vi "CRYImp wiz p4 curve select.vi"(6 "x-y settings array":T1 {"yp db ref" format="%.2f"; "ym db ref" format="%.2f"; "x db ref" format="%.2f"}, 8 "error in (no error)":errorcluster, 9 "Data in":string[][](array[string]), 10 "Main info cluster":T3, 11 "Page flags":T2) -> (0 "error out":errorcluster, 1 "Data out":string[][](array[string]), 2 "Main info cluster out":T3, 3 "Page flags out":T2, 4 "x-y settings array out":T1 {"yp db ref" format="%.2f"; "ym db ref" format="%.2f"; "x db ref" format="%.2f"}, 5 "Data array out":string[](array[string]))   [LabVIEW 2013]
uses:
  Control/CRYImp wiz page flags.ctl
  Control/CRYImp wiz main info.ctl
  Control/CRYx-y settings array.ctl
  CRYImp wiz global.vi
  CRYMainGlobal.vi
panel:
  in  "add":bool
  in  "remove":bool
  in  "apply def":bool
  in  "Curves":i32(listbox) caption="曲线"
  in  "finish b":bool
  in  "cancel 2":bool
  out "table":string[][](table)
  out "cancel":bool
  in  "yp db ref":dbl=1.0
  in  "yp unit":string="deg."
  in  "yp prefix":u16(ring)=8 items=["E", "P", "T", "G", "M", "k", "h", "da", "", "d", "c", "m", "µ", "n", "p", "f", "a"]
  in  "yp axis type":u16(ring)=1 items=["log", "linear"]
  in  "yp data type":u16(ring) caption="aaaa" items=["dB", "linear"]
  in  "ym db ref":dbl
  in  "ym unit":string
  in  "ym prefix":u16(ring)=8 items=["E", "P", "T", "G", "M", "k", "h", "da", "", "d", "c", "m", "µ", "n", "p", "f", "a"]
  in  "ym axis type":u16(ring) items=["log", "linear"]
  in  "ym data type":u16(ring) caption="大小" items=["dB", "linear"]
  in  "x db ref":dbl=1.0 caption="db ref 水平"
  in  "x Unit":string caption="单位"
  in  "x Unit Prefix":u16(ring)=8 caption="单位前缀" items=["E", "P", "T", "G", "M", "k", "h", "da", "", "d", "c", "m", "µ", "n", "p", "f", "a"]
  in  "x Axis type":u16(ring) caption="轴类型" items=["log", "linear"]
  in  "x Data type":u16(ring) caption="数据类型" items=["dB", "linear"]
  in  "Name:":string caption="名字:"
  in  "x col":i32=1 caption="行/列:" min=1
  in  "phase incl":bool caption="相位行/列包括"
  in  "y col":i32=1 caption="行/列:" min=1
  in  "cont":bool
  in  "prev":bool
  in  "next":bool
  in  "X axis:":i32(slide)
  in  "Y axis:":i32(slide)
  in  "Data increment:":i32=1 caption="columns" min=1
  in  "X axis starting column:":i32=1 min=1
  in  "Y axis starting column:":i32=2 min=1
  in  "update":bool
  in  "save setgs":bool
  out "X-Y data series layout":bool
  out "Y axis settings":bool caption="Y轴设置"
  out "X axis settings":bool caption="X轴设置"
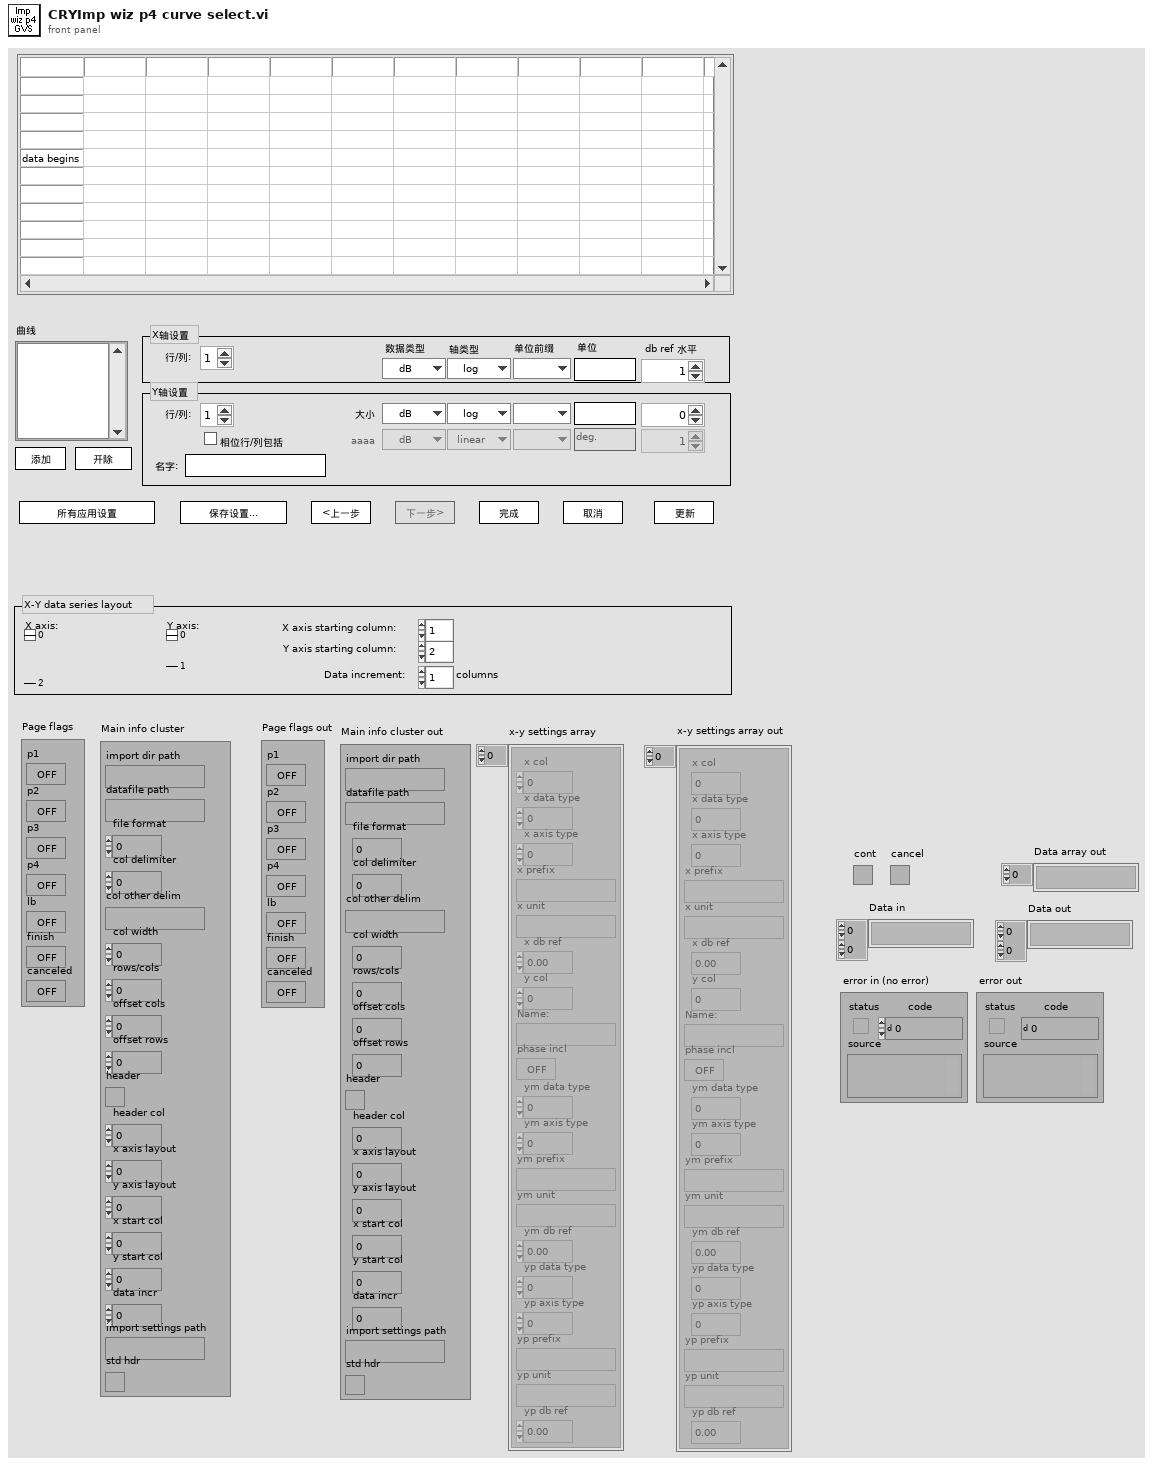
[diagram p1: front panel]
types:
  T1 = typedef "CRYx-y settings array.ctl" = cluster{"x col":i32, "x data type":u16, "x axis type":u16, "x prefix":string, "x unit":string, "x db ref":dbl, "y col":i32, "Name:":string, "phase incl":bool, "ym data type":u16, "ym axis type":u16, "ym prefix":string, "ym unit":string, "ym db ref":dbl, "yp data type":u16, "yp axis type":u16, "yp prefix":string, "yp unit":string, "yp db ref":dbl}[]
  T2 = typedef "CRYImp wiz page flags.ctl" = cluster{"p1":bool, "p2":bool, "p3":bool, "p4":bool, "lb":bool, "finish":bool, "canceled":bool}
  T3 = typedef "CRYImp wiz main info.ctl" = cluster{"import dir path":path, "datafile path":path, "file format":i32, "col delimiter":i32, "col other delim":string, "col width":i32, "rows/cols":i32, "offset cols":i32, "offset rows":i32, "header":bool, "header col":i32, "x axis layout":i32, "y axis layout":i32, "x start col":i32, "y start col":i32, "data incr":i32, "import settings path":path, "std hdr":bool}
  T4 = cluster{"x col":i32, "x data type":u16, "x axis type":u16, "x prefix":string, "x unit":string, "x db ref":dbl, "y col":i32, "Name:":string, "phase incl":bool, "ym data type":u16, "ym axis type":u16, "ym prefix":string, "ym unit":string, "ym db ref":dbl, "yp data type":u16, "yp axis type":u16, "yp prefix":string, "yp unit":string, "yp db ref":dbl}
  T5 = enum16{"open", "open or create", "create or replace", "create"}
  T6 = cluster{"next":bool, "prev":bool, "add":bool, "remove":bool, "apply def":bool, "Curves":i32, "finish b":bool, "cancel 2":bool, "X axis:":i32, "Y axis:":i32, "X axis starting column:":i32, "Y axis starting column:":i32, "Data increment:":i32, "update":bool, "save setgs":bool, "finish":bool}
  T7 = cluster{"x col":i32, "x data type":u16, "x axis type":u16, "x prefix":string, "x unit":string, "x db ref":dbl, "y col":i32, "Name:":string, "phase incl":bool, "ym data type":u16, "ym axis type":u16, "ym prefix":string, "ym unit":string, "ym db ref":dbl, "yp data type":u16, "yp axis type":u16, "yp prefix":string, "yp unit":string, "yp db ref":dbl}[]
  T8 = cluster{"x col":i32, "x data type":u16, "x axis type":u16, "x prefix":string, "x unit":string, "x db ref":dbl}
  T9 = typedef "CRYData Cluster.ctl" = cluster{"Name":string, "Curve":cluster{"x":dbl, "y":dbl, "z":dbl}[], "X data":u16, "Y data":u16, "Z data":u16, "X axis":u16, "Y axis":u16, "Z axis":u16, "X unit":string, "Y unit":string, "Z unit":string, "X dB ref":dbl, "Y dB ref":dbl, "Z dB ref":dbl, "single val":bool, "protected":bool, "display X":bool, "display Y":bool, "display Z":bool, "Test Info":string, "Step No.":i32, "Plot Settings":cluster{"Color":u32, "Interpolation":u8, "Point Style":u8, "Line Style":u8, "Point Color":u32, "Line Width":u8, "Bar Plot Style":u8, "Fill To":i16}, "AutoProtect":bool}
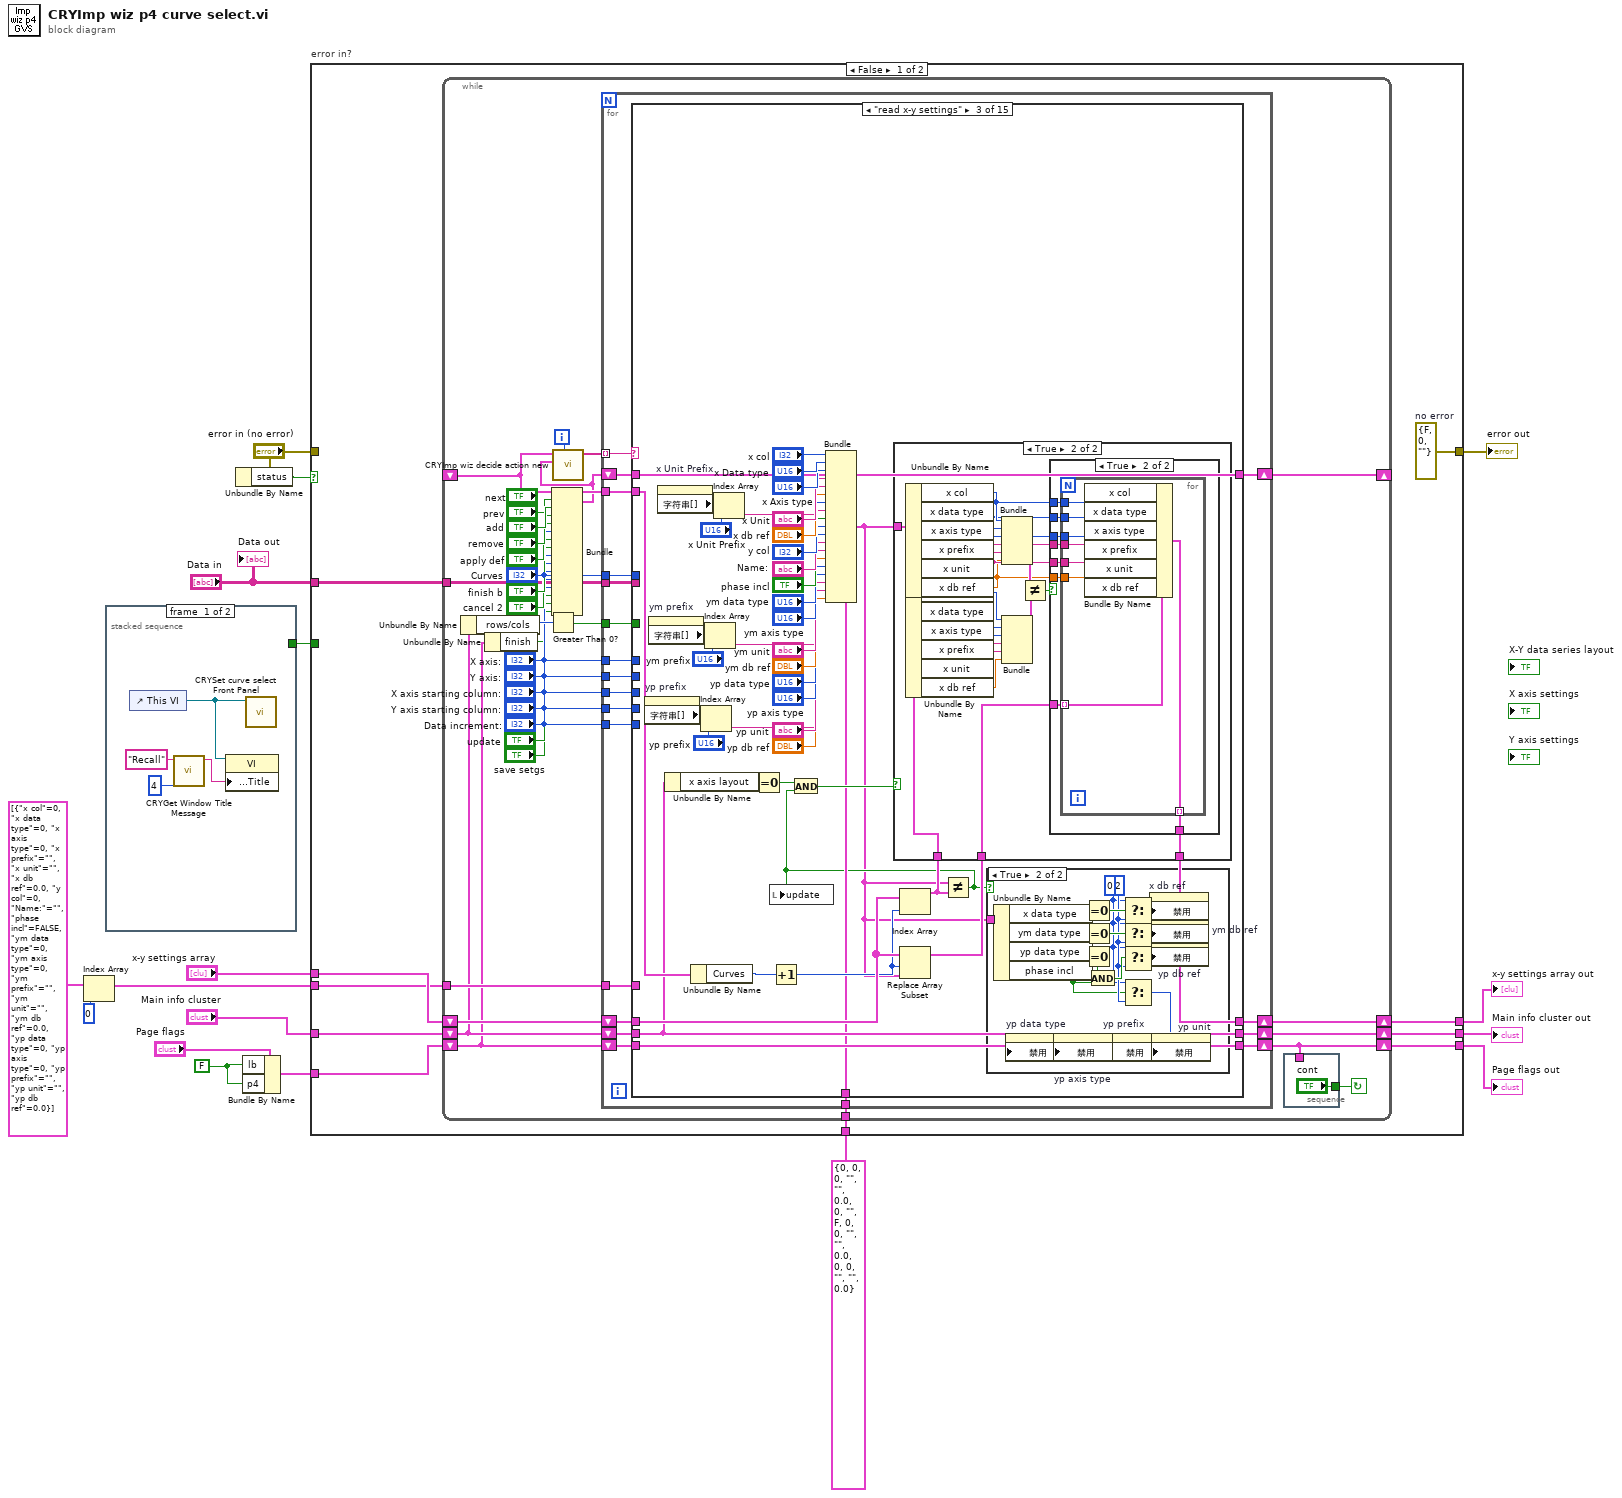
[diagram p0: block diagram]
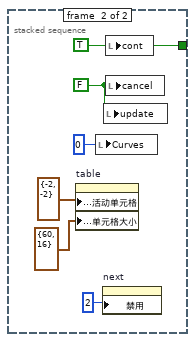
[diagram p2: hidden frame]
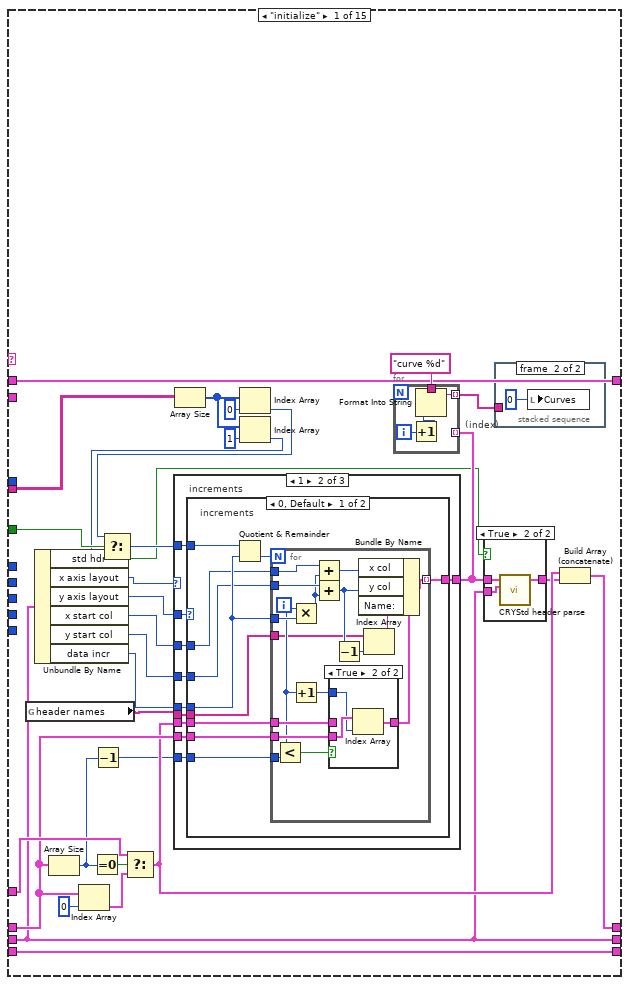
[diagram p3: hidden frame]
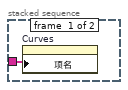
[diagram p5: hidden frame]
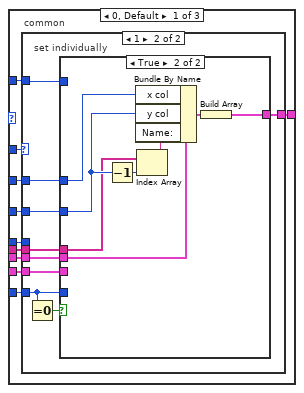
[diagram p6: hidden frame]
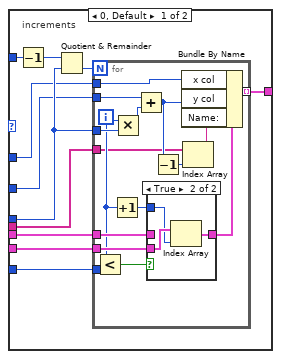
[diagram p7: hidden frame]
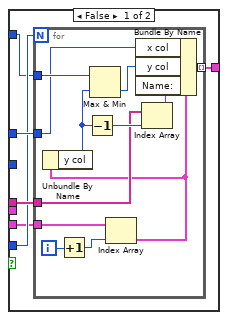
[diagram p9: hidden frame]
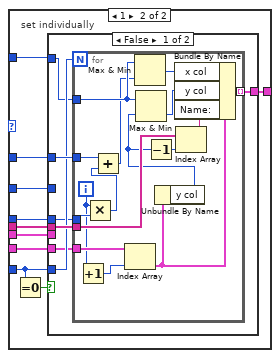
[diagram p11: hidden frame]
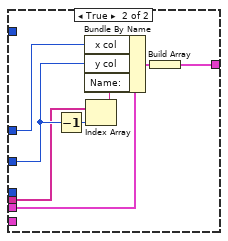
[diagram p12: hidden frame]
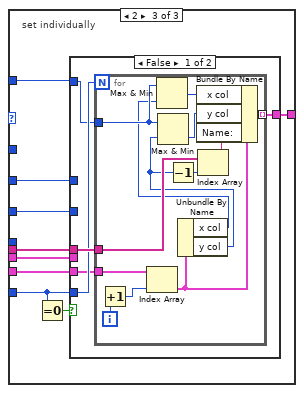
[diagram p13: hidden frame]
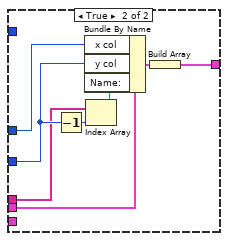
[diagram p14: hidden frame]
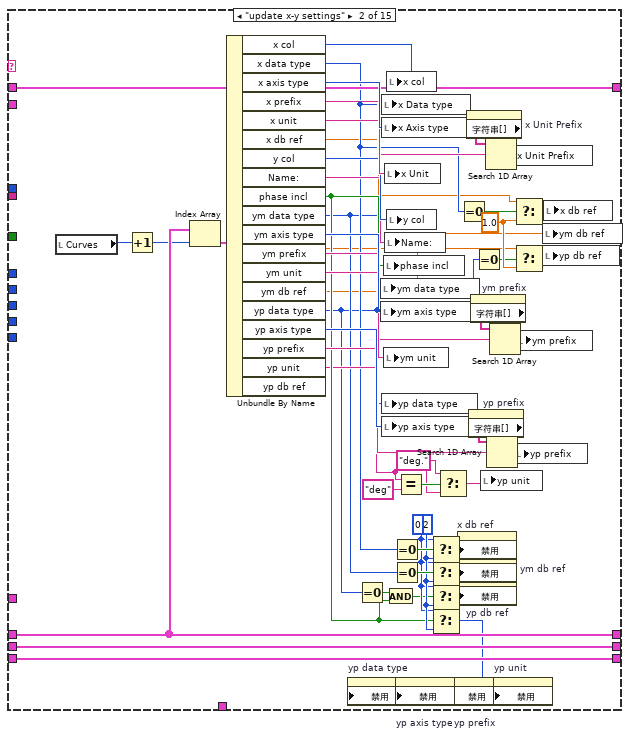
[diagram p15: hidden frame]
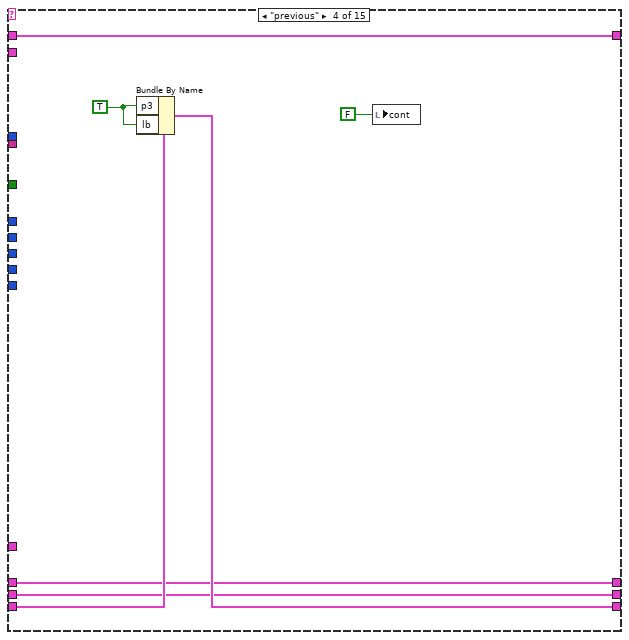
[diagram p19: hidden frame]
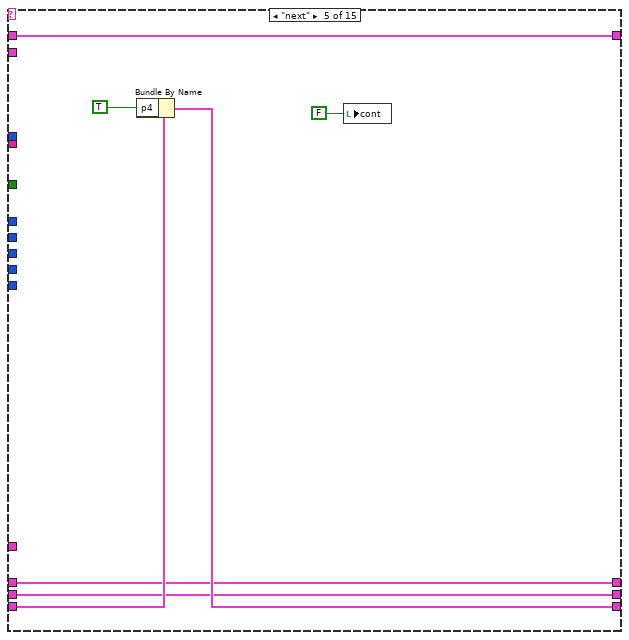
[diagram p20: hidden frame]
diagram:
  w7 = FALSE ("Bundle Element")
  n1 = Index Array(array=T1 [{"x col"=0, "x data type"=0, "x axis type"=0, "x prefix"="", "x unit"="", "x db ref"=0.0, "y col"=0, "Name:"="", "phase incl"=FALSE, "ym data type"=0, "ym axis type"=0, "ym prefix"="", "ym unit"="", "ym db ref"=0.0, "yp data type"=0, "yp axis type"=0, "yp prefix"="", "yp unit"="", "yp db ref"=0.0}] ("x-y settings array"), index=0 ("Dimension Size")) -> (element=w3:T4)
  n2 = stacked-sequence {
    tunnel: [_ w27] -> w17
    frame #0 {
      n3 = control-ref of="This VI"() -> (w19:refnum<vi>)
      n4 = call "CRYGet Window Title Message.vi"("No"=4, "Kind"="Recall") -> ("Multibyte String"=w18:string)  [unwired: 4 in, 5 out]
      n5 = property class="VI"(reference=w19, "Front Panel.Title"=w18) -> ()  [unwired: 1 in, 2 out]
      n6 = call "CRYSet curve select Front Panel.vi"("Vi Ref"=w19) -> ()  [unwired: 11 in]
    }
    frame #1 {
      w23 = FALSE ("cancelled?")
      w27 = TRUE ("cont")
      n7 = property on="table" class="Tbl (strict)"("活动单元格:活动单元格"=cluster{i32, i32} {-2, -2} ("Write Attribute"), "活动单元格:单元格大小"=cluster{"Width":u32, "Height":u32} {"Width"=60, "Height"=16} ("Write Attribute")) -> ()  [unwired: 2 in, 2 out]
      n8 = local write "Curves"(0 ("Data Series")) -> ()
      n9 = property on="next" class="Bool"("禁用"=u8 2 ("Write Attribute")) -> ()  [unwired: 2 in, 2 out]
      n10 = local write "update"(w23) -> ()
      n11 = local write "cont"(w27) -> ()
      n12 = local write "cancel"(w23) -> ()
    }
  }
  n13 = Unbundle By Name("error in (no error)") -> ("status"=w11:bool)
  n14 = Bundle By Name(cluster="Page flags", "lb"=w7, "p4"=w7) -> (w8:T2)
  n15 = case "error in?" shown="False" w11 {
    tunnel: w17 -> [_ _]
    tunnel: "Data in" -> [w37 _]
    tunnel: "Main info cluster" -> [w36 w854]
    tunnel: w8 -> [w35 w853]
    tunnel: [w34 w854] -> w14
    tunnel: [w33 w853] -> w13
    tunnel: "error in (no error)" -> [_ w855]
    tunnel: [w32 w855] -> w10
    tunnel: "x-y settings array" -> [w31 w852]
    tunnel: [w30 w852] -> w5
    tunnel: w3 -> [w29 _]
    tunnel: T4 {"x col"=0, "x data type"=0, "x axis type"=0, "x prefix"="", "x unit"="", "x db ref"=0.0, "y col"=0, "Name:"="", "phase incl"=FALSE, "ym data type"=0, "ym axis type"=0, "ym prefix"="", "ym unit"="", "ym db ref"=0.0, "yp data type"=0, "yp axis type"=0, "yp prefix"="", "yp unit"="", "yp db ref"=0.0} ("Output Element") -> [w28 _]
    frame False {
      w32 = errorcluster {"status"=FALSE, "code"=0, "source"=""}  # no error
      n16 = while {
        tunnel: w28 -> [w38]
        shift-left: w35 -> [w42]
        shift-right: [w48] -> w33
        shift-left: w36 -> [w52]
        shift-right: [w56] -> w34
        tunnel: w29 -> [w59]
        shift-left: w31 -> [w62]
        shift-right: [w49] -> w30
        shift-left: _ -> [w60]
        shift-right: [w50] -> _
        tunnel: w37 -> [w63]
        i -> [w65]
        stop <- w57 continue-if-true
        n17 = Unbundle By Name(w52) -> ("rows/cols"=w53:i32)
        n18 = Unbundle By Name(w42) -> ("finish"=w39:bool)
        n19 = Greater Than 0?(x=w53) -> (x > 0?=w58:bool)
        n20 = Bundle("next"="next", "prev"="prev", "add"="add", "remove"="remove", "apply def"="apply def", "Curves"="Curves", "finish b"="finish b", "cancel 2"="cancel 2", "X axis:"="X axis:", "Y axis:"="Y axis:", "X axis starting column:"="X axis starting column:", "Y axis starting column:"="Y axis starting column:", "Data increment:"="Data increment:", "update"="update", "save setgs"="save setgs", "finish"=w39) -> (w51:T6)  [unwired: 1 out]
        n21 = call "CRYImp wiz decide action new.vi"("Iteration"=w65, "New controls"=w51, "Old controls"=w60) -> ("Frames to run"=w64:string[])  [unwired: 8 in]
        n22 = for {
          tunnel: w64 -> [w91] mode=indexing
          tunnel: w63 -> [w90]
          shift-right: [w89] -> w49
          shift-left: w62 -> [w88]
          tunnel: "Curves" -> [w87]
          tunnel: w58 -> [w86]
          tunnel: w60 -> [w85]
          tunnel: w59 -> [w84]
          shift-right: [w81] -> w56
          shift-left: w52 -> [w83]
          shift-right: [w80] -> w48
          shift-left: w42 -> [w82]
          shift-right: [w78] -> w50
          shift-left: w51 -> [w79]
          tunnel: "X axis:" -> [w77]
          tunnel: "Y axis:" -> [w76]
          tunnel: "X axis starting column:" -> [w75]
          tunnel: "Y axis starting column:" -> [w74]
          tunnel: "Data increment:" -> [w73]
          tunnel: w38 -> [w72]
          n23 = case shown="\"read x-y settings\"" w91 {
            tunnel: w90 -> [w93 _ _ _ _ _ w500 _ _ _ _ _ _ w775 _]
            tunnel: [w114 w368 w389 w472 w480 w487 w503 w621 w629 w644 w669 w693 w731 w767 w851] -> w89
            tunnel: w88 -> [w108 w368 w397 w472 w480 w487 w503 w621 w623 w646 w676 w701 w731 w767 w851]
            tunnel: w87 -> [_ _ _ _ _ _ _ _ w625 _ w667 _ _ _ _]
            tunnel: w86 -> [w117 _ _ _ _ _ w504 _ _ _ _ _ _ _ _]
            tunnel: w85 -> [_ _ w401 _ _ _ _ _ _ _ _ w700 _ _ _]
            tunnel: w84 -> [w110 _ _ _ _ _ _ _ _ _ _ _ _ _ _]
            tunnel: w83 -> [w94 w366 w394 w473 w481 w488 w499 w618 w628 w643 w671 w708 w724 w766 w849]
            tunnel: w82 -> [w113 w365 w400 w475 w483 w490 w498 w616 w627 w642 w670 w707 w739 w774 w848]
            tunnel: [w94 w366 w394 w473 w481 w488 w499 w618 w628 w643 w671 w708 w719 w766 w849] -> w81
            tunnel: [w113 w365 w400 w474 w482 w489 w498 w615 w627 w642 w670 w707 w739 w774 w848] -> w80
            tunnel: w79 -> [w112 w363 w399 w470 w477 w484 w497 w614 w626 w648 w664 w709 w740 w776 w847]
            tunnel: [w112 w363 w399 w470 w477 w484 w497 w614 w626 w647 w663 w709 w740 w776 w847] -> w78
            tunnel: w77 -> [_ _ _ _ _ _ _ _ _ _ _ _ _ _ _]
            tunnel: w76 -> [_ _ _ _ _ _ _ _ _ _ _ _ _ _ _]
            tunnel: w75 -> [_ _ _ _ _ _ _ _ _ _ _ w697 _ _ _]
            tunnel: w74 -> [_ _ _ _ _ _ _ _ _ _ _ w696 _ _ _]
            tunnel: w73 -> [_ _ _ _ _ _ _ _ _ _ _ _ _ _ _]
            tunnel: w72 -> [_ _ w379 _ _ _ _ _ _ _ _ _ _ _ _]
            frame "initialize" {
              # "(index)"
              n24 = global read "CRYImp wiz global.vi" "header names"() -> (w92:string[])
              n25 = Unbundle By Name(w94) -> ("std hdr"=w95:bool, "x axis layout"=w104:i32, "y axis layout"=w103:i32, "x start col"=w102:i32, "y start col"=w101:i32, "data incr"=w100:i32)
              n26 = Array Size(array=w108) -> (size(s)=w98:i32)
              n27 = Index Array(array=w108, index=0 ("Index")) -> (element=w107:T4)
              n28 = Equal To 0?(x=w98) -> (x = 0?=w111:bool)
              n29 = Decrement(x=w98) -> (x-1=w99:i32)
              n30 = Select(t=w110, s=w111, f=w107) -> (s? t:f=w106:T4)
              n31 = Array Size(array=w93) -> (size(s)=w120:i32[])
              n32 = Index Array(array=w120, index=0 ("Index")) -> (element=w116:i32)
              n33 = Index Array(array=w120, index=1 ("Index")) -> (element=w115:i32)
              n34 = Select(t=w116, s=w117, f=w115) -> (s? t:f=w119:i32)
              n35 = case shown="1" w104 {
                tunnel: w103 -> [w142 w218 _]
                tunnel: w100 -> [w141 w217 _]
                tunnel: w119 -> [w140 w216 w291]
                tunnel: w106 -> [w139 w215 w294]
                tunnel: [w138 w214 w298] -> w97
                tunnel: w102 -> [w137 w213 w297]
                tunnel: w101 -> [w136 w212 w296]
                tunnel: w108 -> [w135 w211 w295]
                tunnel: w99 -> [w134 w210 w292]
                tunnel: w92 -> [w133 w209 w293]
                frame 0, Default {
                  # "common"
                  n36 = case shown="1" w142 {
                    tunnel: w141 -> [w150 _]
                    tunnel: w140 -> [w144 w174]
                    tunnel: w139 -> [w152 w182]
                    tunnel: [w151 w181] -> w138
                    tunnel: w137 -> [w149 w180]
                    tunnel: w136 -> [w148 w179]
                    tunnel: w135 -> [w147 w175]
                    tunnel: w134 -> [w146 w176]
                    tunnel: w133 -> [w145 w178]
                    frame 0, Default {
                      # "increments"
                      n37 = Decrement(x=w144) -> (x-1=w143:i32)
                      n38 = Quotient & Remainder(x=w143, y=w150) -> (floor(x/y)=w153:i32)  [unwired: 1 out]
                      n39 = for {
                        N: w153 -> [_]
                        tunnel: w152 -> [w161]
                        tunnel: [w169] -> w151 mode=indexing
                        tunnel: w150 -> [w168]
                        tunnel: w149 -> [w166]
                        tunnel: w148 -> [w165]
                        tunnel: w147 -> [w162]
                        tunnel: w146 -> [w164]
                        tunnel: w145 -> [w155]
                        i -> [w158]
                        n40 = Less?(x=w158, y=w164) -> (x < y?=w163:bool)
                        n41 = Increment(x=w158) -> (x+1=w159:i32)
                        n42 = Multiply(x=w158, y=w168) -> (x*y=w167:i32)
                        n43 = Add(x=w165, y=w167) -> (x+y=w156:i32)
                        n44 = case shown="True" w163 {
                          tunnel: w162 -> [_ w173]
                          tunnel: w161 -> [w170 _]
                          tunnel: [w170 w172] -> w160
                          tunnel: w159 -> [_ w171]
                          frame False {
                          }
                          frame True {
                            n45 = Index Array(array=w173, index=w171) -> (element=w172:T4)
                          }
                        }
                        n46 = Decrement(x=w156) -> (x-1=w157:i32)
                        n47 = Index Array(array=w155, index=w157) -> (element=w154:string)
                        n48 = Bundle By Name(cluster=w160, "x col"=w166, "y col"=w156, "Name:"=w154) -> (w169:T4)
                      }
                    }
                    frame 1 {
                      # "set individually"
                      n49 = Equal To 0?(x=w176) -> (x = 0?=w177:bool)
                      n50 = case shown="True" w177 {
                        tunnel: w182 -> [_ w208]
                        tunnel: [w186 w206] -> w181
                        tunnel: w180 -> [w188 w205]
                        tunnel: w179 -> [_ w203]
                        tunnel: w178 -> [w187 w202]
                        tunnel: w174 -> [w184 _]
                        tunnel: w176 -> [w185 _]
                        tunnel: w175 -> [w183 _]
                        frame False {
                          n51 = for {
                            N: w185 -> [_]
                            tunnel: w188 -> [w194]
                            tunnel: w187 -> [w199]
                            tunnel: [w197] -> w186 mode=indexing
                            tunnel: w184 -> [w195]
                            tunnel: w183 -> [w190]
                            i -> [w192]
                            n52 = Increment(x=w192) -> (x+1=w191:i32)
                            n53 = Index Array(array=w190, index=w191) -> (element=w189:T4)
                            n54 = Unbundle By Name(w189) -> ("y col"=w193:i32)
                            n55 = Decrement(x=w193) -> (x-1=w200:i32)
                            n56 = Max & Min(x=w195, y=w193) -> (min(x,y)=w196:i32)  [unwired: 1 out]
                            n57 = Index Array(array=w199, index=w200) -> (element=w198:string)
                            n58 = Bundle By Name(cluster=w189, "x col"=w194, "y col"=w196, "Name:"=w198) -> (w197:T4)
                          }
                        }
                        frame True {
                          n59 = Decrement(x=w203) -> (x-1=w204:i32)
                          n60 = Index Array(array=w202, index=w204) -> (element=w201:string)
                          n61 = Bundle By Name(cluster=w208, "x col"=w205, "y col"=w203, "Name:"=w201) -> (w207:T4)
                          n62 = Build Array(w207) -> (w206:T7)
                        }
                      }
                    }
                  }
                }
                frame 1 {
                  # "increments"
                  n63 = case shown="0, Default" w218 {
                    tunnel: w217 -> [w225 w252]
                    tunnel: w216 -> [w222 w250]
                    tunnel: w215 -> [w227 w255]
                    tunnel: [w226 w253] -> w214
                    tunnel: w213 -> [w224 w258]
                    tunnel: w212 -> [w223 w257]
                    tunnel: w211 -> [w221 w251]
                    tunnel: w210 -> [w220 w254]
                    tunnel: w209 -> [w219 w256]
                    frame 0, Default {
                      # "increments"
                      n64 = Quotient & Remainder(x=w222, y=w225) -> (floor(x/y)=w228:i32)  [unwired: 1 out]
                      n65 = for {
                        N: w228 -> [_]
                        tunnel: w227 -> [w238]
                        tunnel: [w245] -> w226 mode=indexing
                        tunnel: w225 -> [w244]
                        tunnel: w224 -> [w242]
                        tunnel: w223 -> [w243]
                        tunnel: w221 -> [w237]
                        tunnel: w220 -> [w236]
                        tunnel: w219 -> [w230]
                        i -> [w234]
                        n66 = Less?(x=w234, y=w236) -> (x < y?=w239:bool)
                        n67 = Multiply(x=w234, y=w244) -> (x*y=w241:i32)
                        n68 = Increment(x=w234) -> (x+1=w233:i32)
                        n69 = Add(x=w242, y=w241) -> (x+y=w240:i32)
                        n70 = Add(x=w243, y=w241) -> (x+y=w232:i32)
                        n71 = case shown="True" w239 {
                          tunnel: w237 -> [_ w249]
                          tunnel: w238 -> [w246 _]
                          tunnel: [w246 w248] -> w235
                          tunnel: w233 -> [_ w247]
                          frame False {
                          }
                          frame True {
                            n72 = Index Array(array=w249, index=w247) -> (element=w248:T4)
                          }
                        }
                        n73 = Decrement(x=w232) -> (x-1=w231:i32)
                        n74 = Index Array(array=w230, index=w231) -> (element=w229:string)
                        n75 = Bundle By Name(cluster=w235, "x col"=w240, "y col"=w232, "Name:"=w229) -> (w245:T4)
                      }
                    }
                    frame 1 {
                      # "set individually"
                      n76 = Equal To 0?(x=w254) -> (x = 0?=w259:bool)
                      n77 = case shown="False" w259 {
                        tunnel: w255 -> [_ w290]
                        tunnel: [w264 w288] -> w253
                        tunnel: w258 -> [w266 w287]
                        tunnel: w257 -> [_ w285]
                        tunnel: w256 -> [w265 w284]
                        tunnel: w250 -> [w262 _]
                        tunnel: w254 -> [w263 _]
                        tunnel: w252 -> [w261 _]
                        tunnel: w251 -> [w260 _]
                        frame False {
                          n78 = for {
                            N: w263 -> [_]
                            tunnel: w266 -> [w273]
                            tunnel: w265 -> [w281]
                            tunnel: [w279] -> w264 mode=indexing
                            tunnel: w262 -> [w276]
                            tunnel: w261 -> [w275]
                            tunnel: w260 -> [w270]
                            i -> [w267]
                            n79 = Increment(x=w267) -> (x+1=w271:i32)
                            n80 = Multiply(x=w267, y=w275) -> (x*y=w274:i32)
                            n81 = Add(x=w273, y=w274) -> (x+y=w272:i32)
                            n82 = Index Array(array=w270, index=w271) -> (element=w269:T4)
                            n83 = Max & Min(x=w276, y=w272) -> (min(x,y)=w278:i32)  [unwired: 1 out]
                            n84 = Unbundle By Name(w269) -> ("y col"=w268:i32)
                            n85 = Max & Min(x=w276, y=w268) -> (min(x,y)=w277:i32)  [unwired: 1 out]
                            n86 = Decrement(x=w268) -> (x-1=w282:i32)
                            n87 = Index Array(array=w281, index=w282) -> (element=w280:string)
                            n88 = Bundle By Name(cluster=w269, "x col"=w278, "y col"=w277, "Name:"=w280) -> (w279:T4)
                          }
                        }
                        frame True {
                          n89 = Decrement(x=w285) -> (x-1=w286:i32)
                          n90 = Index Array(array=w284, index=w286) -> (element=w283:string)
                          n91 = Bundle By Name(cluster=w290, "x col"=w287, "y col"=w285, "Name:"=w283) -> (w289:T4)
                          n92 = Build Array(w289) -> (w288:T7)
                        }
                      }
                    }
                  }
                }
                frame 2 {
                  # "set individually"
                  n93 = Equal To 0?(x=w292) -> (x = 0?=w299:bool)
                  n94 = case shown="False" w299 {
                    tunnel: w294 -> [_ w325]
                    tunnel: [w303 w323] -> w298
                    tunnel: w297 -> [_ w322]
                    tunnel: w296 -> [_ w320]
                    tunnel: w293 -> [w304 w319]
                    tunnel: w291 -> [w301 _]
                    tunnel: w292 -> [w302 _]
                    tunnel: w295 -> [w300 _]
                    frame False {
                      n95 = for {
                        N: w302 -> [_]
                        tunnel: w304 -> [w316]
                        tunnel: [w314] -> w303 mode=indexing
                        tunnel: w301 -> [w311]
                        tunnel: w300 -> [w308]
                        i -> [w309]
                        n96 = Increment(x=w309) -> (x+1=w310:i32)
                        n97 = Index Array(array=w308, index=w310) -> (element=w307:T4)
                        n98 = Unbundle By Name(w307) -> ("x col"=w305:i32, "y col"=w306:i32)
                        n99 = Max & Min(x=w311, y=w305) -> (min(x,y)=w313:i32)  [unwired: 1 out]
                        n100 = Max & Min(x=w311, y=w306) -> (min(x,y)=w312:i32)  [unwired: 1 out]
                        n101 = Decrement(x=w306) -> (x-1=w317:i32)
                        n102 = Index Array(array=w316, index=w317) -> (element=w315:string)
                        n103 = Bundle By Name(cluster=w307, "x col"=w313, "y col"=w312, "Name:"=w315) -> (w314:T4)
                      }
                    }
                    frame True {
                      n104 = Decrement(x=w320) -> (x-1=w321:i32)
                      n105 = Index Array(array=w319, index=w321) -> (element=w318:string)
                      n106 = Bundle By Name(cluster=w325, "x col"=w322, "y col"=w320, "Name:"=w318) -> (w324:T4)
                      n107 = Build Array(w324) -> (w323:T7)
                    }
                  }
                }
              }
              n108 = for {
                tunnel: "curve %d" -> [w130]
                tunnel: [w129] -> w105 mode=indexing
                tunnel: w97 -> [_] mode=indexing
                i -> [w132]
                n109 = Increment(x=w132) -> (x+1=w131:i32)
                n110 = Format Into String(format string=w130, w131) -> (resulting string=w129:string)  [unwired: 2 in, 1 out]
              }
              n111 = case shown="True" w95 {
                tunnel: [w123 w124] -> w96
                tunnel: w97 -> [w123 w126]
                tunnel: w94 -> [_ w125]
                frame False {
                }
                frame True {
                  n112 = call "CRYStd header parse.vi"("Main info cluster"=w125, "x-y settings array"=w126) -> ("x-y settings array out"=w124:T1)  [unwired: 9 in]
                }
              }
              n113 = stacked-sequence {
                tunnel: w105 -> [w127 _]
                frame #0 {
                  n114 = property on="Curves" class="LstBox (strict)"("项名"=w127) -> ()  [unwired: 2 in, 2 out]
                }
                frame #1 {
                  n115 = local write "Curves"(0 ("Data Series")) -> ()
                }
              }
              n116 = Build Array (concatenate)(w106, w96) -> (w114:T1)
            }
            frame "update x-y settings" {
              w331 = 1.0 ("x db ref")
              w347 = u8 2 ("Write Attribute")
              w346 = u8 0 ("Write Attribute")
              n117 = local read "Curves"() -> (w364:i32)
              n118 = Increment(x=w364) -> (x+1=w362:i32)
              n119 = Index Array(array=w368, index=w362) -> (element=w367:T4)
              n120 = Unbundle By Name(w367) -> ("x col"=w376:i32, "x data type"=w336:u16, "x axis type"=w375:u16, "x prefix"=w361:string, "x unit"=w374:string, "x db ref"=w334:dbl, "y col"=w373:i32, "Name:"=w372:string, "phase incl"=w344:bool, "ym data type"=w332:u16, "ym axis type"=w371:u16, "ym prefix"=w360:string, "ym unit"=w370:string, "ym db ref"=w326:dbl, "yp data type"=w329:u16, "yp axis type"=w369:u16, "yp prefix"=w359:string, "yp unit"=w339:string, "yp db ref"=w327:dbl)
              n121 = Equal To 0?(x=w329) -> (x = 0?=w343:bool)
              n122 = local write "ym data type"(w332) -> ()
              n123 = local write "ym axis type"(w371) -> ()
              n124 = local write "x Data type"(w336) -> ()
              n125 = local write "x Axis type"(w375) -> ()
              n126 = local write "yp data type"(w329) -> ()
              n127 = local write "yp axis type"(w369) -> ()
              n128 = local write "phase incl"(w344) -> ()
              n129 = local write "ym unit"(w370) -> ()
              n130 = local write "x Unit"(w374) -> ()
              n131 = local write "Name:"(w372) -> ()
              n132 = And(x=w343, y=w344) -> (x .and. y?=w342:bool)
              n133 = local write "x col"(w376) -> ()
              n134 = local write "y col"(w373) -> ()
              n135 = Equal To 0?(x=w336) -> (x = 0?=w352:bool)
              n136 = Equal To 0?(x=w332) -> (x = 0?=w351:bool)
              n137 = Equal?(x=w339, y="deg") -> (x = y?=w340:bool)
              n138 = Select(t=w346, s=w352, f=w347) -> (s? t:f=w350:u8)
              n139 = Select(t=w346, s=w351, f=w347) -> (s? t:f=w349:u8)
              n140 = Select(t=w346, s=w342, f=w347) -> (s? t:f=w348:u8)
              n141 = Select(t=w346, s=w344, f=w347) -> (s? t:f=w345:u8)
              n142 = property on="yp data type" class="Ring (strict)"("禁用"=w345) -> ()  [unwired: 2 in, 2 out]
              n143 = property on="yp axis type" class="Ring (strict)"("禁用"=w345) -> ()  [unwired: 2 in, 2 out]
              n144 = Select(t="deg." ("y"), s=w340, f=w339) -> (s? t:f=w338:string)
              n145 = property on="yp prefix" class="Ring (strict)"("禁用"=w345) -> ()  [unwired: 2 in, 2 out]
              n146 = property on="x db ref" class="DigNum (strict)"("禁用"=w350) -> ()  [unwired: 2 in, 2 out]
              n147 = property on="ym db ref" class="DigNum (strict)"("禁用"=w349) -> ()  [unwired: 2 in, 2 out]
              n148 = property on="yp db ref" class="DigNum (strict)"("禁用"=w348) -> ()  [unwired: 2 in, 2 out]
              n149 = Equal To 0?(x=w336) -> (x = 0?=w335:bool)
              n150 = property on="x Unit Prefix" class="Ring (strict)"() -> ("字符串[]"=w354:string[])  [unwired: 2 in, 2 out]
              n151 = property on="yp prefix" class="Ring (strict)"() -> ("字符串[]"=w356:string[])  [unwired: 2 in, 2 out]
              n152 = property on="ym prefix" class="Ring (strict)"() -> ("字符串[]"=w358:string[])  [unwired: 2 in, 2 out]
              n153 = Equal To 0?(x=w329) -> (x = 0?=w330:bool)
              n154 = local write "yp unit"(w338) -> ()
              n155 = Search 1D Array(1D array=w354, element=w361) -> (index of element=w353:i32)  [unwired: 1 out]
              n156 = Search 1D Array(1D array=w356, element=w359) -> (index of element=w355:i32)  [unwired: 1 out]
              n157 = Search 1D Array(1D array=w358, element=w360) -> (index of element=w357:i32)  [unwired: 1 out]
              n158 = property on="yp unit" class="Str"("禁用"=w345) -> ()  [unwired: 2 in, 2 out]
              n159 = local write "x Unit Prefix"(w353) -> ()
              n160 = Select(t=w334, s=w335, f=w331) -> (s? t:f=w333:dbl)
              n161 = Select(t=w327, s=w330, f=w331) -> (s? t:f=w328:dbl)
              n162 = local write "yp prefix"(w355) -> ()
              n163 = local write "ym prefix"(w357) -> ()
              n164 = local write "ym db ref"(w326) -> ()
              n165 = local write "yp db ref"(w328) -> ()
              n166 = local write "x db ref"(w333) -> ()
            }
            frame "read x-y settings" {
              n167 = property on="yp prefix" class="Ring (strict)"() -> ("字符串[]"=w384:string[])  [unwired: 2 in, 2 out]
              n168 = property on="ym prefix" class="Ring (strict)"() -> ("字符串[]"=w386:string[])  [unwired: 2 in, 2 out]
              n169 = property on="x Unit Prefix" class="Ring (strict)"() -> ("字符串[]"=w388:string[])  [unwired: 2 in, 2 out]
              n170 = Unbundle By Name(w394) -> ("x axis layout"=w395:i32)
              n171 = Unbundle By Name(w401) -> ("Curves"=w398:i32)
              n172 = Index Array(array=w384, index="yp prefix") -> (element=w380:string)
              n173 = Index Array(array=w386, index="ym prefix") -> (element=w381:string)
              n174 = Index Array(array=w388, index="x Unit Prefix") -> (element=w382:string)
              n175 = Equal To 0?(x=w395) -> (x = 0?=w393:bool)
              n176 = Increment(x=w398) -> (x+1=w396:i32)
              n177 = Bundle(cluster=w379, "x col"="x col", "x data type"="x Data type", "x axis type"="x Axis type", "x prefix"=w382, "x unit"="x Unit", "x db ref"="x db ref", "y col"="y col", "Name:"="Name:", "phase incl"="phase incl", "ym data type"="ym data type", "ym axis type"="ym axis type", "ym prefix"=w381, "ym unit"="ym unit", "ym db ref"="ym db ref", "yp data type"="yp data type", "yp axis type"="yp axis type", "yp prefix"=w380, "yp unit"="yp unit", "yp db ref"="yp db ref") -> (w377:T4)
              n178 = Index Array(array=w397, index=w396) -> (element=w390:T4)
              n179 = Replace Array Subset(array=w397, new element=w377, index=w396) -> (w391:T1)
              n180 = Not Equal?(x=w377, y=w390) -> (x != y?=w378:bool)
              n181 = local write "update"(w378) -> ()
              n182 = And(x=w393, y=w378) -> (x .and. y?=w392:bool)
              n183 = case shown="True" w392 {
                tunnel: w391 -> [w433 w442]
                tunnel: w390 -> [_ w452]
                tunnel: w377 -> [_ w451]
                tunnel: [w433 w441] -> w389
                frame False {
                }
                frame True {
                  n184 = Unbundle By Name(w451) -> ("x col"=w439:i32, "x data type"=w438:u16, "x axis type"=w437:u16, "x prefix"=w436:string, "x unit"=w435:string, "x db ref"=w434:dbl)
                  n185 = Unbundle By Name(w452) -> ("x col"=w445:i32, "x data type"=w446:u16, "x axis type"=w450:u16, "x prefix"=w449:string, "x unit"=w448:string, "x db ref"=w447:dbl)
                  n186 = Bundle("x col"=w439, "x data type"=w438, "x axis type"=w437, "x prefix"=w436, "x unit"=w435, "x db ref"=w434) -> (w444:T8)  [unwired: 1 out]
                  n187 = Bundle("x col"=w445, "x data type"=w446, "x axis type"=w450, "x prefix"=w449, "x unit"=w448, "x db ref"=w447) -> (w443:T8)  [unwired: 1 out]
                  n188 = Not Equal?(x=w444, y=w443) -> (x != y?=w440:bool)
                  n189 = case shown="True" w440 {
                    tunnel: w442 -> [w453 w461]
                    tunnel: [w453 w460] -> w441
                    tunnel: w439 -> [_ w459]
                    tunnel: w438 -> [_ w458]
                    tunnel: w437 -> [_ w457]
                    tunnel: w436 -> [_ w456]
                    tunnel: w435 -> [_ w455]
                    tunnel: w434 -> [_ w454]
                    frame False {
                    }
                    frame True {
                      n190 = for {
                        tunnel: w461 -> [w469] mode=indexing
                        tunnel: [w468] -> w460 mode=indexing
                        tunnel: w459 -> [w467]
                        tunnel: w458 -> [w466]
                        tunnel: w457 -> [w465]
                        tunnel: w456 -> [w464]
                        tunnel: w455 -> [w463]
                        tunnel: w454 -> [w462]
                        n191 = Bundle By Name(cluster=w469, "x col"=w467, "x data type"=w466, "x axis type"=w465, "x prefix"=w464, "x unit"=w463, "x db ref"=w462) -> (w468:T4)
                      }
                    }
                  }
                }
              }
              n192 = case shown="True" w378 {
                tunnel: w377 -> [_ w432]
                frame False {
                }
                frame True {
                  w421 = u8 2 ("Write Attribute")
                  w419 = u8 0 ("Write Attribute")
                  n193 = Unbundle By Name(w432) -> ("x data type"=w431:u16, "ym data type"=w429:u16, "yp data type"=w430:u16, "phase incl"=w420:bool)
                  n194 = Equal To 0?(x=w431) -> (x = 0?=w428:bool)
                  n195 = Equal To 0?(x=w429) -> (x = 0?=w427:bool)
                  n196 = Equal To 0?(x=w430) -> (x = 0?=w423:bool)
                  n197 = And(x=w423, y=w420) -> (x .and. y?=w422:bool)
                  n198 = Select(t=w419, s=w428, f=w421) -> (s? t:f=w426:u8)
                  n199 = Select(t=w419, s=w427, f=w421) -> (s? t:f=w425:u8)
                  n200 = Select(t=w419, s=w422, f=w421) -> (s? t:f=w424:u8)
                  n201 = Select(t=w419, s=w420, f=w421) -> (s? t:f=w418:u8)
                  n202 = property on="yp data type" class="Ring (strict)"("禁用"=w418) -> ()  [unwired: 2 in, 2 out]
                  n203 = property on="yp axis type" class="Ring (strict)"("禁用"=w418) -> ()  [unwired: 2 in, 2 out]
                  n204 = property on="yp prefix" class="Ring (strict)"("禁用"=w418) -> ()  [unwired: 2 in, 2 out]
                  n205 = property on="x db ref" class="DigNum (strict)"("禁用"=w426) -> ()  [unwired: 2 in, 2 out]
                  n206 = property on="ym db ref" class="DigNum (strict)"("禁用"=w425) -> ()  [unwired: 2 in, 2 out]
                  n207 = property on="yp db ref" class="DigNum (strict)"("禁用"=w424) -> ()  [unwired: 2 in, 2 out]
                  n208 = property on="yp unit" class="Str"("禁用"=w418) -> ()  [unwired: 2 in, 2 out]
                }
              }
            }
            frame "previous" {
              w476 = TRUE ("Bundle Element")
              n209 = Bundle By Name(cluster=w475, "p3"=w476, "lb"=w476) -> (w474:T2)
              n210 = local write "cont"(FALSE ("cont")) -> ()
            }
            frame "next" {
              n211 = Bundle By Name(cluster=w483, "p4"=TRUE ("Bundle Element")) -> (w482:T2)
              n212 = local write "cont"(FALSE ("cont")) -> ()
            }
            frame "finish" {
              w486 = TRUE ("Bundle Element")
              n213 = Bundle By Name(cluster=w490, "p4"=w486, "finish"=w486) -> (w489:T2)
              n214 = local write "cont"(FALSE ("cont")) -> ()
            }
            frame "data array make" {
              n215 = call "CRYUnflatten Data.vi"() -> ("Datum"=w505:T9)  [unwired: 9 in, 2 out]
              n216 = Array Subset(array=w503, index=1 ("Array Index")) -> (w502:T1)  [unwired: 1 in]
              n217 = for {
                tunnel: w502 -> [w577] mode=indexing
                tunnel: w505 -> [w576]
                tunnel: w504 -> [w575]
                tunnel: w500 -> [w574]
                tunnel: [w562] -> w492 mode=indexing
                i -> [w558]
                w526 = u16 0 items=["dB", "linear"] ("ym data type")
                w540 = u16 0 items=["dB", "linear"] ("ym data type")
                w551 = u16 0 items=["dB", "linear"] ("ym data type")
                n218 = local read "x Data type"() -> (w525:u16)
                n219 = local read "yp data type"() -> (w539:u16)
                n220 = Unbundle By Name(w577) -> ("x col"=w572:i32, "x data type"=w569:u16, "x axis type"=w567:u16, "x unit"=w523:string, "x db ref"=w511:dbl, "y col"=w571:i32, "Name:"=w557:string, "phase incl"=w573:bool, "ym data type"=w568:u16, "ym axis type"=w566:u16, "ym unit"=w542:string, "ym db ref"=w509:dbl, "yp data type"=w565:u16, "yp axis type"=w564:u16, "yp unit"=w533:string, "yp db ref"=w507:dbl)
                n221 = local read "ym data type"() -> (w550:u16)
                n222 = call "CRYString all white space.vi"("String"=w557) -> ("Nothing but white space?"=w559:bool)  [unwired: 10 in]
                n223 = local read "x Unit Prefix"() -> (w512:u16)
                n224 = case shown="True" w559 {
                  tunnel: w558 -> [_ w583]
                  tunnel: w557 -> [w578 _]
                  tunnel: [w578 w579] -> w556
                  frame False {
                  }
                  frame True {
                    n225 = Increment(x=w583) -> (x+1=w582:i32)
                    n226 = Format Into String(format string="%d", initial string="curve ", w582) -> (resulting string=w579:string)  [unwired: 1 in, 1 out]
                  }
                }
                n227 = local read "ym prefix"() -> (w514:u16)
                n228 = local read "yp prefix"() -> (w515:u16)
                n229 = property on="ym prefix" class="Ring (strict)"() -> ("Strings []"=w513:string[])  [unwired: 2 in, 2 out]
                n230 = Equal?(x=w525, y=w526) -> (x = y?=w524:bool)
                n231 = Decrement(x=w572) -> (x-1=w561:i32)
                n232 = Equal?(x=w539, y=w540) -> (x = y?=w538:bool)
                n233 = Decrement(x=w571) -> (x-1=w560:i32)
                n234 = Equal?(x=w550, y=w551) -> (x = y?=w549:bool)
                n235 = Index Array(array=w513, index=w512) -> (element=w516:string)
                n236 = Index Array(array=w513, index=w514) -> (element=w517:string)
                n237 = Index Array(array=w513, index=w515) -> (element=w518:string)
                n238 = Increment(x=w560) -> (x+1=w570:i32)
                n239 = case shown="True" w575 {
                  tunnel: w574 -> [w592 w607]
                  tunnel: w573 -> [w591 w606]
                  tunnel: w561 -> [w590 w601]
                  tunnel: w560 -> [w589 w600]
                  tunnel: w570 -> [w588 w599]
                  tunnel: [w585 w603] -> w554
                  tunnel: [w587 w605] -> w555
                  tunnel: [w586 w604] -> w553
                  frame True {
                    n240 = Index Array(array=w592, index (row)=w590) -> (element=w585:string[])  [unwired: 1 in]
                    n241 = Index Array(array=w592, index (row)=w589) -> (element=w587:string[])  [unwired: 1 in]
                    n242 = Array Size(array=w585) -> (size(s)=w584:i32)
                    n243 = case shown="True" w591 {
                      tunnel: w592 -> [_ w598]
                      tunnel: w588 -> [_ w597]
                      tunnel: [w593 w596] -> w586
                      tunnel: w584 -> [w595 _]
                      frame False {
                        n244 = Initialize Array("0.0", w595) -> (w593:string[])
                      }
                      frame True {
                        n245 = Index Array(array=w598, index (row)=w597) -> (element=w596:string[])  [unwired: 1 in]
                      }
                    }
                  }
                  frame False {
                    n246 = Index Array(array=w607, index (col)=w601) -> (element=w603:string[])  [unwired: 1 in]
                    n247 = Index Array(array=w607, index (col)=w600) -> (element=w605:string[])  [unwired: 1 in]
                    n248 = Array Size(array=w603) -> (size(s)=w602:i32)
                    n249 = case shown="False" w606 {
                      tunnel: w607 -> [_ w613]
                      tunnel: [w608 w612] -> w604
                      tunnel: w602 -> [w610 _]
                      tunnel: w599 -> [_ w611]
                      frame False {
                        n250 = Initialize Array("0.0", w610) -> (w608:string[])
                      }
                      frame True {
                        n251 = Index Array(array=w613, index (col)=w611) -> (element=w612:string[])  [unwired: 1 in]
                      }
                    }
                  }
                }
                n252 = call "CRYUnit Prefix to Multiplier.vi"("unit prefix"=w516) -> ("multiplier"=w519:dbl)  [unwired: 4 out]
                n253 = call "CRYUnit Prefix to Multiplier.vi"("unit prefix"=w517) -> ("multiplier"=w520:dbl)  [unwired: 4 out]
                n254 = call "CRYUnit Prefix to Multiplier.vi"("unit prefix"=w518) -> ("multiplier"=w521:dbl)  [unwired: 4 out]
                n255 = Multiply(x=w519, y=w511) -> (x*y=w510:dbl)
                n256 = Format Value(format string="%.0p", value (0)=w510) -> (output string=w529:string)  [unwired: 1 in]
                n257 = Concatenate Strings("dB re " ("string"), w529, " " ("string"), w523) -> (w531:string)
                n258 = Multiply(x=w520, y=w509) -> (x*y=w508:dbl)
                n259 = Format Value(format string="%.0p", value (0)=w508) -> (output string=w544:string)  [unwired: 1 in]
                n260 = Concatenate Strings("dB re " ("string"), w544, " " ("string"), w542) -> (w548:string)
                n261 = Multiply(x=w521, y=w507) -> (x*y=w506:dbl)
                n262 = Format Value(format string="%.0p", value (0)=w506) -> (output string=w536:string)  [unwired: 1 in]
                n263 = Concatenate Strings("dB re " ("string"), w536, " " ("string"), w533) -> (w534:string)
                n264 = Select(t=w531, s=w524, f=w523) -> (s? t:f=w522:string)
                n265 = Select(t=w548, s=w549, f=w542) -> (s? t:f=w546:string)
                n266 = Select(t=w534, s=w538, f=w533) -> (s? t:f=w532:string)
                n267 = call "CRYImp wiz curve construct.vi"("Z strings"=w553, "Y strings"=w555, "X strings"=w554) -> ("Curve"=w552:cluster{"x":dbl, "y":dbl, "z":dbl}[])  [unwired: 8 in]
                n268 = Bundle By Name(cluster=w576, "Name"=w556, "Curve"=w552, "X data"=w569, "Y data"=w568, "Z data"=w565, "X axis"=w567, "Y axis"=w566, "Z axis"=w564, "X unit"=w522, "Y unit"=w546, "Z unit"=w532, "X dB ref"=w510, "Y dB ref"=w508, "Z dB ref"=w506) -> (w563:T9)
                n269 = call "CRYFlatten Data.vi"("Datum"=w563) -> ("Data flattened"=w562:string)  [unwired: 10 in]
              }
              "Data array out" <- w492
              n270 = local write "update"(FALSE ("update")) -> ()
              n271 = call "CRYExport data to tab-delimited.vi"("suppress file output (false)"=TRUE, "data series"=w492) -> ("tab-delimited output string"=w495:string)  [unwired: 7 in, 2 out]
              n272 = Spreadsheet String To Array(format string="%s", spreadsheet string=w495, array type (2D Dbl)=string[][] []) -> ()  [unwired: 2 out]
            }
            frame "cancel" {
              n273 = local write "cont"(FALSE ("cont")) -> ()
              n274 = Bundle By Name(cluster=w616, "canceled"=TRUE ("Bundle Element")) -> (w615:T2)
              "cancel" <- TRUE ("cancelled?")
            }
            frame "defaults apply" {
              n275 = Increment(x=w625) -> (x+1=w624:i32)
              n276 = Index Array(array=w623, index=w624) -> (element=w622:T4)
              n277 = Array Subset(array=w623, index=1 ("Array Index")) -> (w631:T1)  [unwired: 1 in]
              n278 = for {
                tunnel: w631 -> [w641] mode=indexing
                tunnel: w622 -> [w637]
                tunnel: [w638] -> w630 mode=indexing
                n279 = Unbundle By Name(w641) -> ("x col"=w640:i32, "y col"=w639:i32, "Name:"=w634:string)
                n280 = Unbundle By Name(w637) -> ("Name:"=w636:string)
                n281 = call "CRYString all white space.vi"("String"=w634) -> ("Nothing but white space?"=w633:bool)  [unwired: 10 in]
                n282 = Select(t=w636, s=w633, f=w634) -> (s? t:f=w635:string)
                n283 = Bundle By Name(cluster=w637, "x col"=w640, "y col"=w639, "Name:"=w635) -> (w638:T4)
              }
              n284 = Build Array (concatenate)(w622, w630) -> (w629:T7)
            }
            frame "add series" {
              n285 = Index Array(array=w646, index=0 ("Index")) -> (element=w649:T4)
              n286 = Build Array (concatenate)(w646, w649) -> (w644:T1)
              n287 = Array Size(array=w646) -> (size(s)=w645:i32)
              n288 = stacked-sequence {
                tunnel: w645 -> [w651 w661]
                tunnel: w648 -> [_ w660]
                tunnel: [_ w659] -> w647
                frame #0 {
                  n289 = for {
                    N: w651 -> [_]
                    tunnel: "curve %d" -> [w655]
                    tunnel: [w654] -> w652 mode=indexing
                    i -> [w657]
                    n290 = Increment(x=w657) -> (x+1=w656:i32)
                    n291 = Format Into String(format string=w655, w656) -> (resulting string=w654:string)  [unwired: 2 in, 1 out]
                  }
                  n292 = property on="Curves" class="LstBox (strict)"("项名"=w652) -> ()  [unwired: 2 in, 2 out]
                }
                frame #1 {
                  n293 = Decrement(x=w661) -> (x-1=w658:i32)
                  n294 = local write "Curves"(w658) -> ()
                  n295 = Bundle By Name(cluster=w660, "Curves"=w658) -> (w659:T6)
                }
              }
            }
            frame "remove series" {
              n296 = Increment(x=w667) -> (x+1=w662:i32)
              n297 = Split 1D Array(array=w676, index=w662) -> (first subarray=w673:T1, second subarray=w674:T1)
              n298 = Array Subset(array=w674, index=1 ("Array Index")) -> (w672:T1)  [unwired: 1 in]
              n299 = Build Array (concatenate)(w673, w672) -> (w669:T1)
              n300 = Array Size(array=w669) -> (size(s)=w668:i32)
              n301 = Decrement(x=w668) -> (x-1=w665:i32)
              n302 = Equal?(x=w668, y=w662) -> (x = y?=w666:bool)
              n303 = stacked-sequence {
                tunnel: w666 -> [_ w687]
                tunnel: w665 -> [w678 w686]
                tunnel: w664 -> [_ w685]
                tunnel: [_ w684] -> w663
                frame #0 {
                  n304 = for {
                    N: w678 -> [_]
                    tunnel: "curve %d" -> [w681]
                    tunnel: [w680] -> w677 mode=indexing
                    i -> [w683]
                    n305 = Increment(x=w683) -> (x+1=w682:i32)
                    n306 = Format Into String(format string=w681, w682) -> (resulting string=w680:string)  [unwired: 2 in, 1 out]
                  }
                  n307 = property on="Curves" class="LstBox (strict)"("项名"=w677) -> ()  [unwired: 2 in, 2 out]
                }
                frame #1 {
                  n308 = case shown="True" w687 {
                    tunnel: w686 -> [_ w692]
                    tunnel: w685 -> [w688 w691]
                    tunnel: [w688 w690] -> w684
                    frame False {
                    }
                    frame True {
                      n309 = Decrement(x=w692) -> (x-1=w689:i32)
                      n310 = local write "Curves"(w689) -> ()
                      n311 = Bundle By Name(cluster=w691, "Curves"=w689) -> (w690:T6)
                    }
                  }
                }
              }
            }
            frame "col shift" {
              n312 = Unbundle By Name(w700) -> ("X axis starting column:"=w699:i32, "Y axis starting column:"=w698:i32)
              n313 = Subtract(x=w697, y=w699) -> (x-y=w695:i32)
              n314 = Subtract(x=w696, y=w698) -> (x-y=w694:i32)
              n315 = Index Array(array=w701, index=0 ("Index")) -> (element=w702:T4)
              n316 = Array Subset(array=w701, index=1 ("Array Index")) -> (w704:T1)  [unwired: 1 in]
              n317 = for {
                tunnel: w704 -> [w712] mode=indexing
                tunnel: [w717] -> w703 mode=indexing
                tunnel: w695 -> [w711]
                tunnel: w694 -> [w710]
                n318 = Unbundle By Name(w712) -> ("x col"=w716:i32, "y col"=w715:i32)
                n319 = Add(x=w716, y=w711) -> (x+y=w714:i32)
                n320 = Add(x=w715, y=w710) -> (x+y=w713:i32)
                n321 = Bundle By Name(cluster=w712, "x col"=w714, "y col"=w713) -> (w717:T4)
              }
              n322 = Build Array (concatenate)(w702, w703) -> (w693:T7)
            }
            frame "save settings" {
              # "add default name here\n(last settings file opened)"
              n323 = Unbundle By Name(w724) -> ("import settings path"=w723:path)
              n324 = global read "CRYMainGlobal.vi" "top path"() -> (w718:path)
              n325 = Build Path(base path=w718, name or relative path="Settings") -> (appended path=w727:path)
              n326 = Strip Path(path=w723) -> (name=w722:string)  [unwired: 1 out]
              n327 = File/Directory Info(path=w727) -> (directory=w728:bool, error out=w730:errorcluster)  [unwired: 1 in, 5 out]
              n328 = Unbundle By Name(w730) -> ("status"=w729:bool)
              n329 = call "CRYStrip step extension.vi"("Step name w/ extension"=w722) -> ("Step name (base)"=w721:string)  [unwired: 7 in, 3 out]
              n330 = Compound Arithmetic op=AND(w728, invert w729) -> (w726:bool)
              n331 = case shown="False" w726 {
                tunnel: w727 -> [w742 w743]
                tunnel: [w741 w743] -> w725
                frame False {
                  n332 = Create Folder(path (use dialog)=w742) -> (created path=w741:path)  [unwired: 1 in, 3 out]
                }
                frame True {
                }
              }
              n333 = call <vilib>:"Open_Create_Replace File.vi"("pattern"="*.imp", "default name"=w721, "prompt"="Enter filename to save", "function (open:0)"=T5."create or replace", "start path  (Not A Path)"=w725) -> ("error out"=w736:errorcluster, "new file path"=w720:path, "refnum"=w735:refnum<file>)  [unwired: 2 in, 2 out]
              n334 = Unbundle By Name(w736) -> ("status"=w737:bool)
              n335 = case shown="False" w737 {
                tunnel: w735 -> [w763 _]
                tunnel: w736 -> [w761 _]
                tunnel: w724 -> [w751 w764]
                tunnel: w731 -> [w753 _]
                tunnel: w720 -> [w750 _]
                tunnel: [w749 w764] -> w719
                frame False {
                  n336 = Bundle By Name(cluster=w751, "import settings path"=w750) -> (w749:T3)
                  n337 = Write to Binary File(file (use dialog)=w763, data=w749, error in=w761, 5:FALSE ("预置数组或字符串大小？(T)")) -> (refnum out=w758:refnum<file>, error out=w757:errorcluster)  [unwired: 3 out]
                  n338 = Bundle("x-y settings array"=w753) -> (w752:cluster{"x-y settings array":T1})  [unwired: 1 in]
                  n339 = Write to Binary File(file (use dialog)=w758, data=w752, error in=w757, 5:FALSE ("预置数组或字符串大小？(T)")) -> (refnum out=w755:refnum<file>, error out=w756:errorcluster)  [unwired: 3 out]
                  n340 = call <vilib>:"compatCalcOffset.vi"("error in"=w756, "pos mode (0:1)"=enum16{"start", "end", "current"}."current", "refnum"=w755) -> ("error out"=w747:errorcluster, "offset"=w746:i32, "dup refnum"=w745:refnum<file>)  [unwired: 1 in, 5 out]
                  n341 = Set File Size(4:w747, 6:w746, 7:w745) -> (0:w760:errorcluster, 3:w762:refnum<file>)
                  n342 = Close File(refnum=w762, error in=w760) -> (error out=w754:errorcluster)  [unwired: 1 out]
                  n343 = call <vilib>:"Simple Error Handler.vi"("error in (no error)"=w754) -> ()  [unwired: 1 in, 8 out]
                }
                frame True {
                }
              }
            }
            frame "table update" {
              w772 = ""
              w779 = 0 ("Index")
              w765 = FALSE  # (no need for header indicator here)
              n344 = Array Size(array=w775) -> (size(s)=w792:i32[])
              n345 = Unbundle By Name(w766) -> ("rows/cols"=w781:i32, "header col"=w780:i32)  [unwired: 1 out]
              n346 = Index Array(array=w792, index=0 ("Index")) -> (element=w778:i32)
              n347 = Index Array(array=w792, index=1 ("Index")) -> (element=w777:i32)
              n348 = case shown="0, Default" w781 {
                tunnel: w777 -> [w833 _]
                tunnel: w775 -> [w835 w839]
                tunnel: w778 -> [_ w840]
                tunnel: [w834 w837] -> w770
                tunnel: w767 -> [w832 w846]
                tunnel: w766 -> [w831 w845]
                frame 0, Default {
                  n349 = call "CRYHeader x-y settings full.vi"("x-y settings array"=w832, "Main info cluster"=w831, "Row length"=w833) -> ("dB ref row out"=w827:string[], "Axis type row out"=w828:string[], "Data type row out"=w829:string[], "Name row out"=w830:string[])  [unwired: 5 in]
                  n350 = Build Array (concatenate)(w830, w829, w828, w827, w835) -> (w834:string[][])
                }
                frame 1 {
                  n351 = Transpose 2D Array(2D array=w839) -> (transposed array=w838:string[][])
                  n352 = call "CRYHeader x-y settings full.vi"("x-y settings array"=w846, "Main info cluster"=w845, "Row length"=w840) -> ("dB ref row out"=w841:string[], "Axis type row out"=w842:string[], "Data type row out"=w843:string[], "Name row out"=w844:string[])  [unwired: 5 in]
                  n353 = Build Array (concatenate)(w844, w843, w842, w841, w838) -> (w836:string[][])
                  n354 = Transpose 2D Array(2D array=w836) -> (transposed array=w837:string[][])
                }
              }
              "table" <- w770
              n355 = Subtract(x=w778, y=w779) -> (x-y=w784:i32)
              n356 = Subtract(x=w777, y=w779) -> (x-y=w783:i32)
              n357 = for {
                N: w784 -> [_]
                tunnel: "row %d" -> [w824]
                tunnel: [w823] -> w786 mode=indexing
                i -> [w826]
                n358 = Increment(x=w826) -> (x+1=w825:i32)
                n359 = Format Into String(format string=w824, w825) -> (resulting string=w823:string)  [unwired: 2 in, 1 out]
              }
              n360 = for {
                N: w783 -> [_]
                tunnel: "col %d" -> [w820]
                tunnel: [w819] -> w788 mode=indexing
                i -> [w822]
                n361 = Increment(x=w822) -> (x+1=w821:i32)
                n362 = Format Into String(format string=w820, w821) -> (resulting string=w819:string)  [unwired: 2 in, 1 out]
              }
              n363 = Initialize Array(w772, w779) -> (w789:string[])
              n364 = Initialize Array(w772, w779) -> (w787:string[])
              n365 = Initialize Array(w772, 4 ("Dimension Size")) -> (w771:string[])
              n366 = case shown="1" w781 {
                tunnel: [w802 w807] -> w769
                tunnel: [w795 w816] -> w768
                tunnel: w789 -> [w806 w818]
                tunnel: w788 -> [w805 _]
                tunnel: w787 -> [w804 w817]
                tunnel: w786 -> [_ w815]
                tunnel: "data begins" -> [w803 w814]
                tunnel: "header" -> [w800 w812]
                tunnel: w765 -> [w799 w811]
                tunnel: w780 -> [w798 w810]
                tunnel: w771 -> [w797 w809]
                frame 0, Default {
                  n367 = Build Array (concatenate)(w804, w803) -> (w801:string[])
                  n368 = Build Array (concatenate)(w806, w805) -> (w802:string[])
                  n369 = call "CRYArray replace with extend.vi"("Enable (T)"=w799, "Index"=w798, "String element"=w800, "String array"=w801) -> ("String array out"=w796:string[])  [unwired: 7 in]
                  n370 = Build Array (concatenate)(w797, w796) -> (w795:string[])
                }
                frame 1 {
                  n371 = Build Array (concatenate)(w817, w815) -> (w816:string[])
                  n372 = Build Array (concatenate)(w818, w814) -> (w813:string[])
                  n373 = call "CRYArray replace with extend.vi"("Enable (T)"=w811, "Index"=w810, "String element"=w812, "String array"=w813) -> ("String array out"=w808:string[])  [unwired: 7 in]
                  n374 = Build Array (concatenate)(w809, w808) -> (w807:string[])
                }
              }
              n375 = property on="table" class="Tbl (strict)"("行首字符串[]"=w768, "列首字符串[]"=w769) -> ()  [unwired: 2 in, 2 out]
            }
            frame "idle", Default {
              n376 = Wait (ms)(milliseconds to wait=u32 150) -> ()  [unwired: 1 out]
            }
          }
        }
        n377 = stacked-sequence {
          tunnel: ["cont"] -> w57
          tunnel: w48 -> [_]
          frame #0 {
          }
        }
      }
    }
    frame True {
    }
  }
  "Page flags out" <- w13
  "Main info cluster out" <- w14
  "error out" <- w10
  "x-y settings array out" <- w5
  "Data out" <- "Data in"
